vi "FPGA_lock-in_v2.vi"() -> ()   [LabVIEW 2013]
uses:
  <vilib>/eio/EIONode/EIONode.xnode
  FPGA_run-states.ctl
  <vilib>/rvi/DataTransferAndStorage/Container/XNode/niFpgaContainer.xnode
  <vilib>/rvi/FIFO/Fifo_Resource/nirvififoEmulationWrite.vi
  <vilib>/rvi/eio/common/nirviEmuTemplateMethod_errors.vi
  <vilib>/rvi/FIFO/Fifo_Resource/nirvififoEmulationRead.vi
  <vilib>/rvi/Memory/Memory_Emulation/nirvimemoryFastEmulation.vi
  <vilib>/rvi/Memory/Memory_Emulation/nirvimemoryEmulation.vi
panel:
  in  "amplitude":u16=100
  in  "DAC mem adr":u32
  out "pan-chan":u16
  in  "inhibate lock-in":bool=TRUE
  in  "clock divider":i32=20
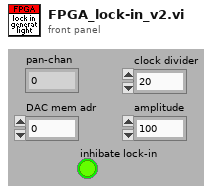
[diagram p1: front panel]
types:
  T1 = typedef "FPGA_run-states.ctl" = enum16{"stopped", "check", "reserve", "run", "release"}
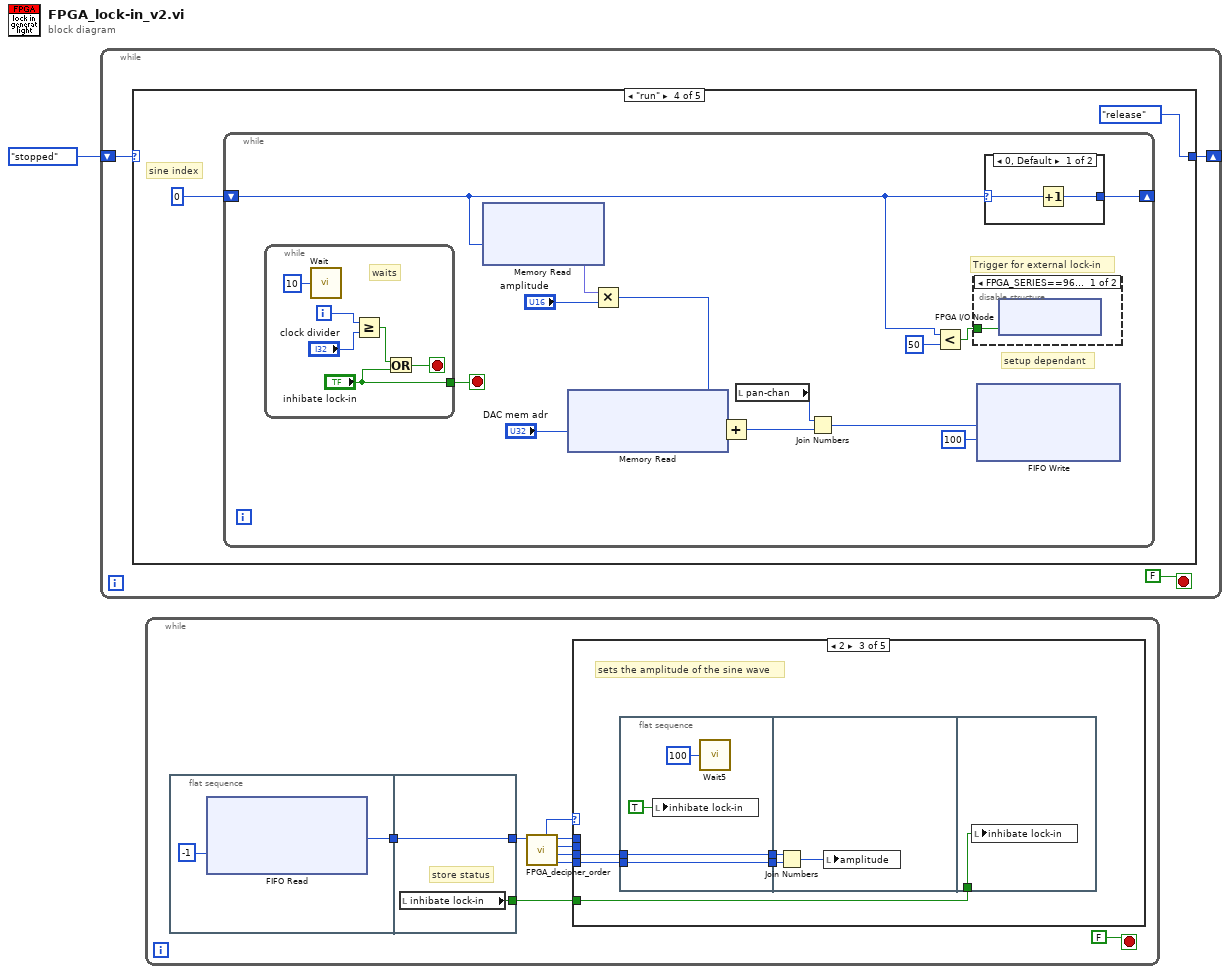
[diagram p0: block diagram]
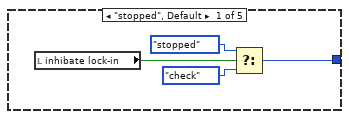
[diagram p2: hidden frame]
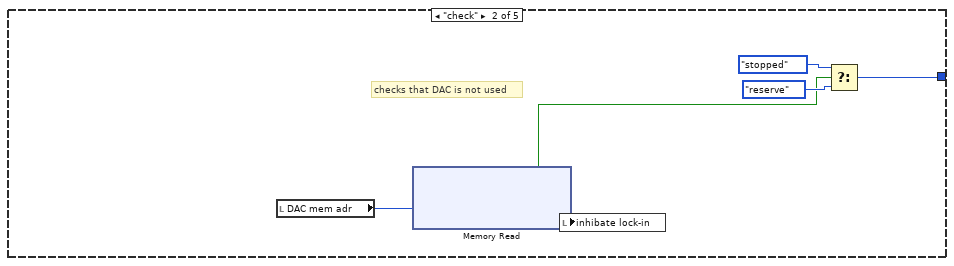
[diagram p3: hidden frame]
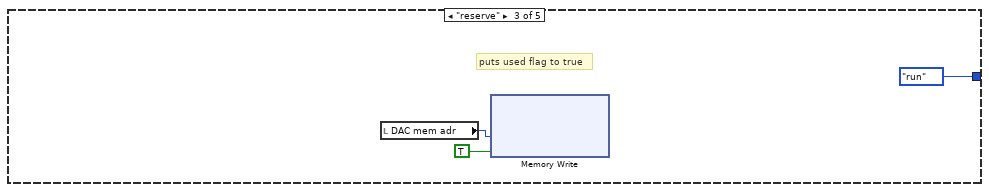
[diagram p4: hidden frame]
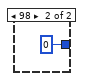
[diagram p5: hidden frame]
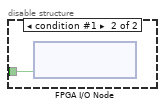
[diagram p6: hidden frame]
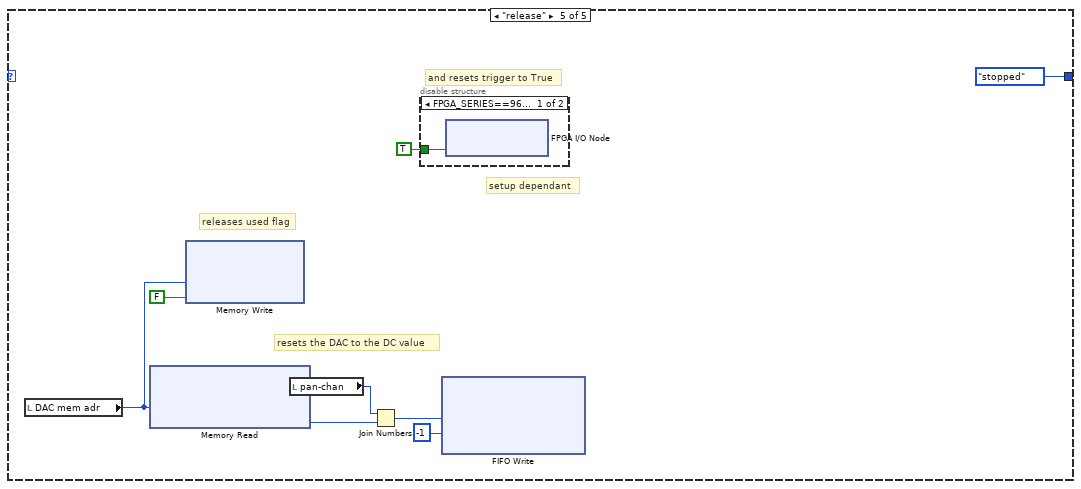
[diagram p7: hidden frame]
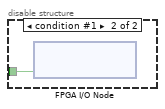
[diagram p8: hidden frame]
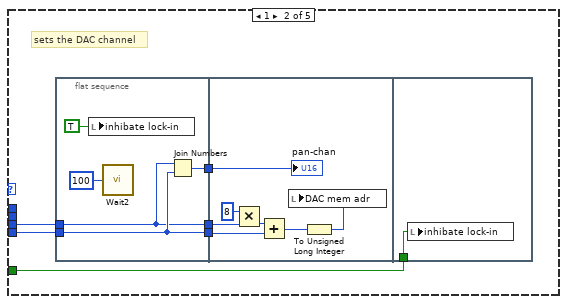
[diagram p10: hidden frame]
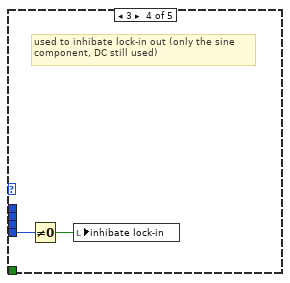
[diagram p11: hidden frame]
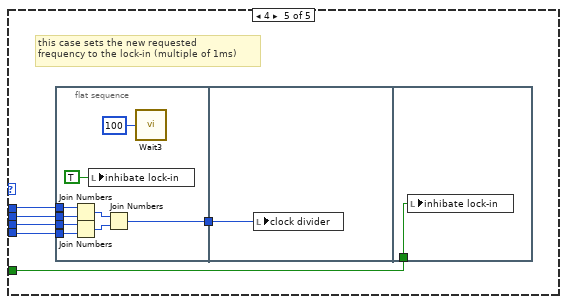
[diagram p12: hidden frame]
diagram:
  n1 = while {
    shift-right: [w3] -> _
    shift-left: FPGA_run-states."stopped" ("run states") -> [w4]
    stop <- FALSE stop-if-true
    n2 = case shown="\"run\"" w4 {
      tunnel: [w5 w10 FPGA_run-states."run" ("run states") FPGA_run-states."release" ("run states") FPGA_run-states."stopped" ("run states")] -> w3
      frame "stopped", Default {
        n3 = local read "inhibate lock-in"() -> (w8:bool)
        n4 = Select(t=FPGA_run-states."stopped" ("run states"), s=w8, f=FPGA_run-states."check" ("run states")) -> (s? t:f=w5:T1)
      }
      frame "check" {
        # "checks that DAC is not used"
        n5 = local read "DAC mem adr"() -> (w13:u32)
        n6 = xnode ("Memory Read")("Address"=w13) -> ("Data"=w9:bool)  [unwired: 1 in, 1 out]
        n7 = local write "inhibate lock-in"(w9) -> ()
        n8 = Select(t=FPGA_run-states."stopped" ("run states"), s=w9, f=FPGA_run-states."reserve" ("run states")) -> (s? t:f=w10:T1)
      }
      frame "reserve" {
        # "puts used flag to true"
        n9 = local read "DAC mem adr"() -> (w16:u32)
        n10 = xnode ("Memory Write")("Address"=w16, "Data"=TRUE) -> ()  [unwired: 1 in, 1 out]
      }
      frame "run" {
        # "sine index"
        n11 = while {
          shift-right: [w23] -> _
          shift-left: u32 0 -> [w21]
          stop <- w26 stop-if-true
          # "setup dependant"
          # "Trigger for external lock-in"
          n12 = while {
            tunnel: ["inhibate lock-in"] -> w26
            i -> [w41]
            stop <- w40 stop-if-true
            # "waits"
            n13 = call "Wait"("Count(uSec)"=u32 10) -> ()  [unwired: 1 out]
            n14 = Greater Or Equal?(x=w41, y="clock divider") -> (x >= y?=w39:bool)
            n15 = Or(x=w39, y="inhibate lock-in") -> (x .or. y?=w40:bool)
          }
          n16 = xnode ("Memory Read")("Address"=w21) -> ("Data"=w28:fxp<+/-,16,1>)  [unwired: 1 in, 1 out]
          n17 = xnode ("Memory Read")("Address"="DAC mem adr") -> ("Data"=w27:u16)  [unwired: 1 in, 1 out]
          n18 = Multiply(x=w28, y="amplitude") -> (x*y=w22:i16)
          n19 = Add(x=w22, y=w27) -> (x+y=w30:u16)
          n20 = local read "pan-chan"() -> (w32:u16)
          n21 = Join Numbers(hi=w32, lo=w30) -> ((hi.lo)=w24:u32)
          n22 = Less?(x=w21, y=u32 50) -> (x < y?=w20:bool)
          n23 = disable-structure shown="FPGA_SERIES==9612, Default" {
            disable-tunnel: w20 -> [w36 w37]
            frame condition #0 (active) {
              n24 = xnode "FPGA I/O Node"("Port0/DIO0"=w36) -> ()  [unwired: 1 in, 1 out]
            }
            frame condition #1 {
              n25 = xnode "FPGA I/O Node"("Port9/DIO0"=w37) -> ()  [unwired: 1 in, 1 out]
            }
          }
          n26 = xnode ("FIFO Write")("Element"=w24, "Timeout"=100) -> ()  [unwired: 1 in, 2 out]
          n27 = case shown="0, Default" w21 {
            selector: w21 -> [w34 _]
            tunnel: [w33 u32 0] -> w23
            frame 0, Default {
              n28 = Increment(x=w34) -> (x+1=w33:u32)
            }
            frame 98 {
            }
          }
        }
      }
      frame "release" {
        # "setup dependant"
        # "and resets trigger to True"
        # "resets the DAC to the DC value"
        # "releases used flag"
        n29 = local read "DAC mem adr"() -> (w49:u32)
        n30 = xnode ("Memory Read")("Address"=w49) -> ("Data"=w47:u16)  [unwired: 1 in, 1 out]
        n31 = xnode ("Memory Write")("Address"=w49, "Data"=FALSE) -> ()  [unwired: 1 in, 1 out]
        n32 = local read "pan-chan"() -> (w50:u16)
        n33 = Join Numbers(hi=w50, lo=w47) -> ((hi.lo)=w46:u32)
        n34 = disable-structure shown="FPGA_SERIES==9612, Default" {
          disable-tunnel: TRUE -> [w52 w53]
          frame condition #0 (active) {
            n35 = xnode "FPGA I/O Node"("Port0/DIO0"=w52) -> ()  [unwired: 1 in, 1 out]
          }
          frame condition #1 {
            n36 = xnode "FPGA I/O Node"("Port9/DIO0"=w53) -> ()  [unwired: 1 in, 1 out]
          }
        }
        n37 = xnode ("FIFO Write")("Element"=w46, "Timeout"=-1) -> ()  [unwired: 1 in, 2 out]
      }
    }
  }
  n38 = while {
    stop <- FALSE stop-if-true
    n39 = flat-sequence {
      tunnel: [w63] -> w55
      tunnel: [w66] -> w61
      tunnel: w55 -> [w66]
      tunnel: [w65] -> w54
      frame #0 {
        n40 = xnode ("FIFO Read")("Timeout"=-1) -> ("Element"=w63:u64)  [unwired: 1 in, 2 out]
      }
      frame #1 {
        # "store status"
        n41 = local read "inhibate lock-in"() -> (w65:bool)
      }
    }
    n42 = call "FPGA_decipher_order.vi"("order in"=w61) -> ("data 1"=w59:u8, "data 2"=w58:u8, "data 3"=w57:u8, "data 4"=w56:u8, "order out"=w60:u8)  [unwired: 6 out]
    n43 = case shown="2" w60 {
      tunnel: w59 -> [_ w71 w89 w100 w102]
      tunnel: w58 -> [_ w72 w90 _ w103]
      tunnel: w57 -> [_ _ _ _ w104]
      tunnel: w56 -> [_ _ _ _ w105]
      tunnel: w54 -> [_ w68 w86 _ w106]
      frame 0, Default {
      }
      frame 1 {
        # "sets the DAC channel"
        n44 = flat-sequence {
          tunnel: [w75] -> w70
          tunnel: [w74] -> w69
          tunnel: w71 -> [w75]
          tunnel: w72 -> [w74]
          tunnel: [w73] -> w67
          tunnel: w70 -> [w80]
          tunnel: w69 -> [w83]
          tunnel: w67 -> [w78]
          tunnel: w68 -> [w85]
          frame #0 {
            n45 = local write "inhibate lock-in"(TRUE ("inhibate lock-in")) -> ()
            n46 = call "Wait2"("Count(uSec)"=u32 100) -> ()  [unwired: 1 out]
            n47 = Join Numbers(hi=w74, lo=w75) -> ((hi.lo)=w73:u16)
          }
          frame #1 {
            n48 = Multiply(x=u8 8, y=w83) -> (x*y=w81:u8)
            n49 = Add(x=w81, y=w80) -> (x+y=w79:u8)
            n50 = To Unsigned Long Integer(number=w79) -> (unsigned 32bit integer=w84:u32)
            n51 = local write "DAC mem adr"(w84) -> ()
            "pan-chan" <- w78
          }
          frame #2 {
            n52 = local write "inhibate lock-in"(w85) -> ()
          }
        }
      }
      frame 2 {
        # "sets the amplitude of the sine wave"
        n53 = flat-sequence {
          tunnel: [w93] -> w88
          tunnel: [w92] -> w87
          tunnel: w89 -> [w93]
          tunnel: w90 -> [w92]
          tunnel: w88 -> [w97]
          tunnel: w87 -> [w96]
          tunnel: w86 -> [w98]
          frame #0 {
            n54 = local write "inhibate lock-in"(TRUE ("inhibate lock-in")) -> ()
            n55 = call "Wait5"("Count(uSec)"=u32 100) -> ()  [unwired: 1 out]
          }
          frame #1 {
            n56 = Join Numbers(hi=w96, lo=w97) -> ((hi.lo)=w95:u16)
            n57 = local write "amplitude"(w95) -> ()
          }
          frame #2 {
            n58 = local write "inhibate lock-in"(w98) -> ()
          }
        }
      }
      frame 3 {
        # "used to inhibate lock-in out (only the sine\ncomponent, DC still used)"
        n59 = Not Equal To 0?(x=w100) -> (x != 0?=w99:bool)
        n60 = local write "inhibate lock-in"(w99) -> ()
      }
      frame 4 {
        # "this case sets the new requested\nfrequency to the lock-in (multiple of 1ms)"
        n61 = flat-sequence {
          tunnel: w105 -> [w111]
          tunnel: w104 -> [w110]
          tunnel: w103 -> [w109]
          tunnel: w102 -> [w108]
          tunnel: [w107] -> w101
          tunnel: w101 -> [w116]
          tunnel: w106 -> [w117]
          frame #0 {
            n62 = Join Numbers(hi=w111, lo=w110) -> ((hi.lo)=w112:u16)
            n63 = Join Numbers(hi=w109, lo=w108) -> ((hi.lo)=w113:u16)
            n64 = local write "inhibate lock-in"(TRUE ("inhibate lock-in")) -> ()
            n65 = Join Numbers(hi=w112, lo=w113) -> ((hi.lo)=w107:u32)
            n66 = call "Wait3"("Count(uSec)"=u32 100) -> ()  [unwired: 1 out]
          }
          frame #1 {
            n67 = local write "clock divider"(w116) -> ()
          }
          frame #2 {
            n68 = local write "inhibate lock-in"(w117) -> ()
          }
        }
      }
    }
  }
